vi "SetDescription.vi"(8 "error in (no error)":errorcluster, 10 "Description":string, 11 "DocumentClass in":refnum<class "Document.lvclass">) -> (0 "error out":errorcluster, 3 "DocumentClass out":refnum<class "Document.lvclass">)   [LabVIEW 2021, in "ProligentXMLGenerator.lvlib" / "Document.lvclass"]
doc: "An optional Description can also be specified."
uses:
  Document.lvclass
  Document.lvclass/Document.ctl
  Base/Attribute/Attribute.lvclass
  Base/NonNullableString_600/NonNullableString_600.lvclass
  C:/Projects/proligent-xml-generator-labview/src/ProligentXMLGenerator/Base/NonNullableString/NonNullableString.lvclass
  C:/Projects/proligent-xml-generator-labview/src/ProligentXMLGenerator/Base/String/String.lvclass
  C:/Projects/proligent-xml-generator-labview/src/ProligentXMLGenerator/Base/Attribute/Attribute.lvclass
  C:/Projects/proligent-xml-generator-labview/src/ProligentXMLGenerator/Base/NonNullableString_600/NonNullableString_600.lvclass
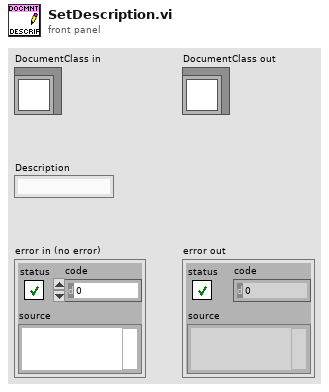
[diagram p1: front panel]
types:
  T1 = typedef "ProligentXMLGenerator.lvlib/Document.lvclass/Data.ctl" = cluster{"Name":string, "CustomData":refnum<class "CustomData.lvclass">, "Identifier":refnum<class "Guid.lvclass">, "NameType":refnum<class "NonEmptyString_255.lvclass">, "FileName":refnum<class "NonEmptyString_255.lvclass">, "Description":refnum<class "NonNullableString_600.lvclass">, "FilePath":path, "DestinationFolder":path}
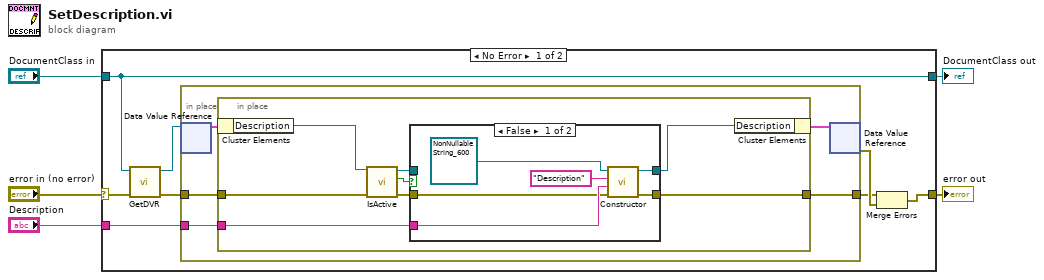
[diagram p0: block diagram]
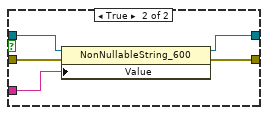
[diagram p2: hidden frame]
diagram:
  n1 = case shown="No Error" "error in (no error)" {
    selector: "error in (no error)" -> [w11 w38]
    tunnel: "DocumentClass in" -> [w6 w39]
    tunnel: [w8 w38] -> w4
    tunnel: "Description" -> [w7 _]
    tunnel: [w6 w39] -> w5
    frame No Error {
      n2 = call "GetDVR.vi"("error in"=w11, "Document in"=w6) -> ("error out"=w10:errorcluster, "DVRReference"=w12:refnum<data-value>)  [unwired: 8 in]
      n3 = in-place "In Place Element Structure" {
        in-place-border: w10 -> [w16]
        in-place-border: [w18] -> w9
        in-place-border: w7 -> [w17]
        n4 = in-place-dvr #1(w12) -> (w15:T1)  [unwired: 1 out]
        n5 = in-place "In Place Element Structure" {
          in-place-border: [w26] -> w18
          in-place-border: w17 -> [w25]
          in-place-border: w16 -> [w24]
          n6 = in-place-cluster #2(w15) -> ("Description"=w20:refnum<class "NonNullableString_600.lvclass">)
          n7 = call "IsActive.vi"("error in"=w24, "Attribute in"=w20) -> ("error out"=w21:errorcluster, "IsActive"=w22:bool, "Attribute in"=w23:refnum<class "NonNullableString_600.lvclass">)  [unwired: 7 in]
          n8 = case shown="False" w22 {
            tunnel: [w29 w37] -> w26
            tunnel: w25 -> [w31 w36]
            tunnel: w23 -> [_ w34]
            tunnel: w21 -> [w30 w35]
            tunnel: [w27 w33] -> w19
            frame False {
              n9 = call-dynamic "Constructor.vi"("error in"=w30, "Value"=w31, "Name"="Description", "String in"=refnum<class "NonNullableString_600.lvclass"> refnum ("IntegrationMetaData")) -> ("error out"=w29:errorcluster, "String out"=w27:refnum<class "NonNullableString_600.lvclass">)  [unwired: 6 in]
            }
            frame True {
              n10 = property on="Property Node" class="NonNullableString_600"(reference=w34, error in=w35, "Value"=w36) -> (reference out=w33:refnum<class "NonNullableString_600.lvclass">, error out=w37:errorcluster)
            }
          }
          n11 = in-place-cluster #2("Description"=w19) -> (w14:T1)
        }
        n12 = in-place-dvr #1(w14) -> (w13:errorcluster)  [unwired: 1 out]
      }
      n13 = Merge Errors(w9, w13) -> (w8:errorcluster)
    }
    frame Error {
    }
  }
  "error out" <- w4
  "DocumentClass out" <- w5
